vi "RunState.TestSockets.MyIndex.vi"(11 "Automation Refnum in":refnum<k7>) -> (3 "Numeric":i32)   [LabVIEW 2020]
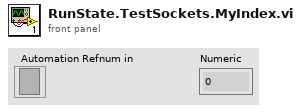
[diagram p1: front panel]
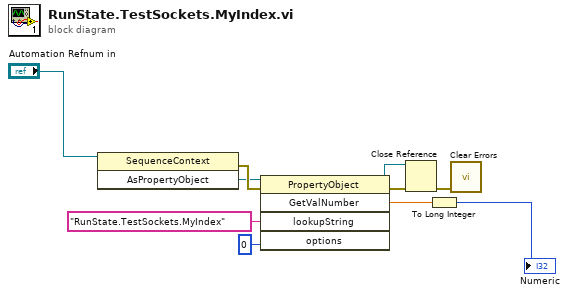
[diagram p0: block diagram]
diagram:
  n1 = invoke class="SequenceContext" method="AsPropertyObject"(reference="Automation Refnum in") -> (error out=w5:errorcluster, "AsPropertyObject"=w1:refnum<k7>)  [unwired: 2 in, 1 out]
  n2 = invoke class="PropertyObject" method="GetValNumber"(reference=w1, error in=w5, "lookupString"="RunState.TestSockets.MyIndex", "options"=0) -> (reference out=w4:refnum<k7>, error out=w3:errorcluster, "GetValNumber"=w7:dbl)  [unwired: 1 in, 2 out]
  n3 = Close Reference(reference=w4, error in (no error)=w3) -> (error out=w6:errorcluster)
  n4 = To Long Integer(number=w7) -> (32bit integer=→"Numeric":i32)
  n5 = call <vilib>:"Clear Errors.vi"("error in (no error)"=w6) -> ()  [unwired: 5 in, 2 out]
